vi "GenericPowerSupply.vi"() -> ()   [LabVIEW 2012]
uses:
  <userlib>/libdriver_powersupply/libdriver_powersupply.lvlib
panel:
  in  "SetCurrent":dbl step=0.2
  in  "ON/OFF":bool
  out "Current":dbl(graph)=10.19439697265625
  out "OPEN":bool
  out "NEG":bool
  out "POS":bool
  out "Alarm":bool
  out "Error":bool
  out "Standby":bool
  out "Operational":bool
  in  "stop":bool
  out "current out":dbl
  in  "Name":string="QUATTEST\u0000"
  in  "MDS":string="mdsserver:5000\u0000"
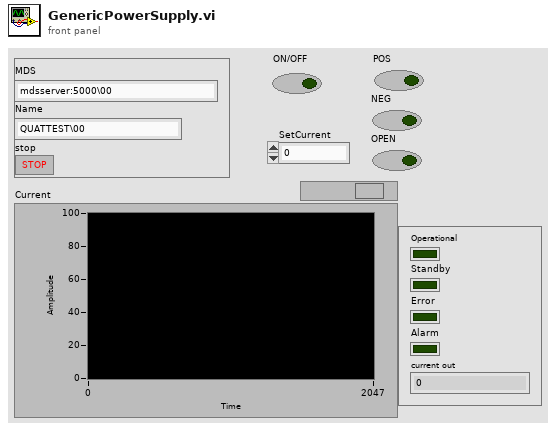
[diagram p1: front panel]
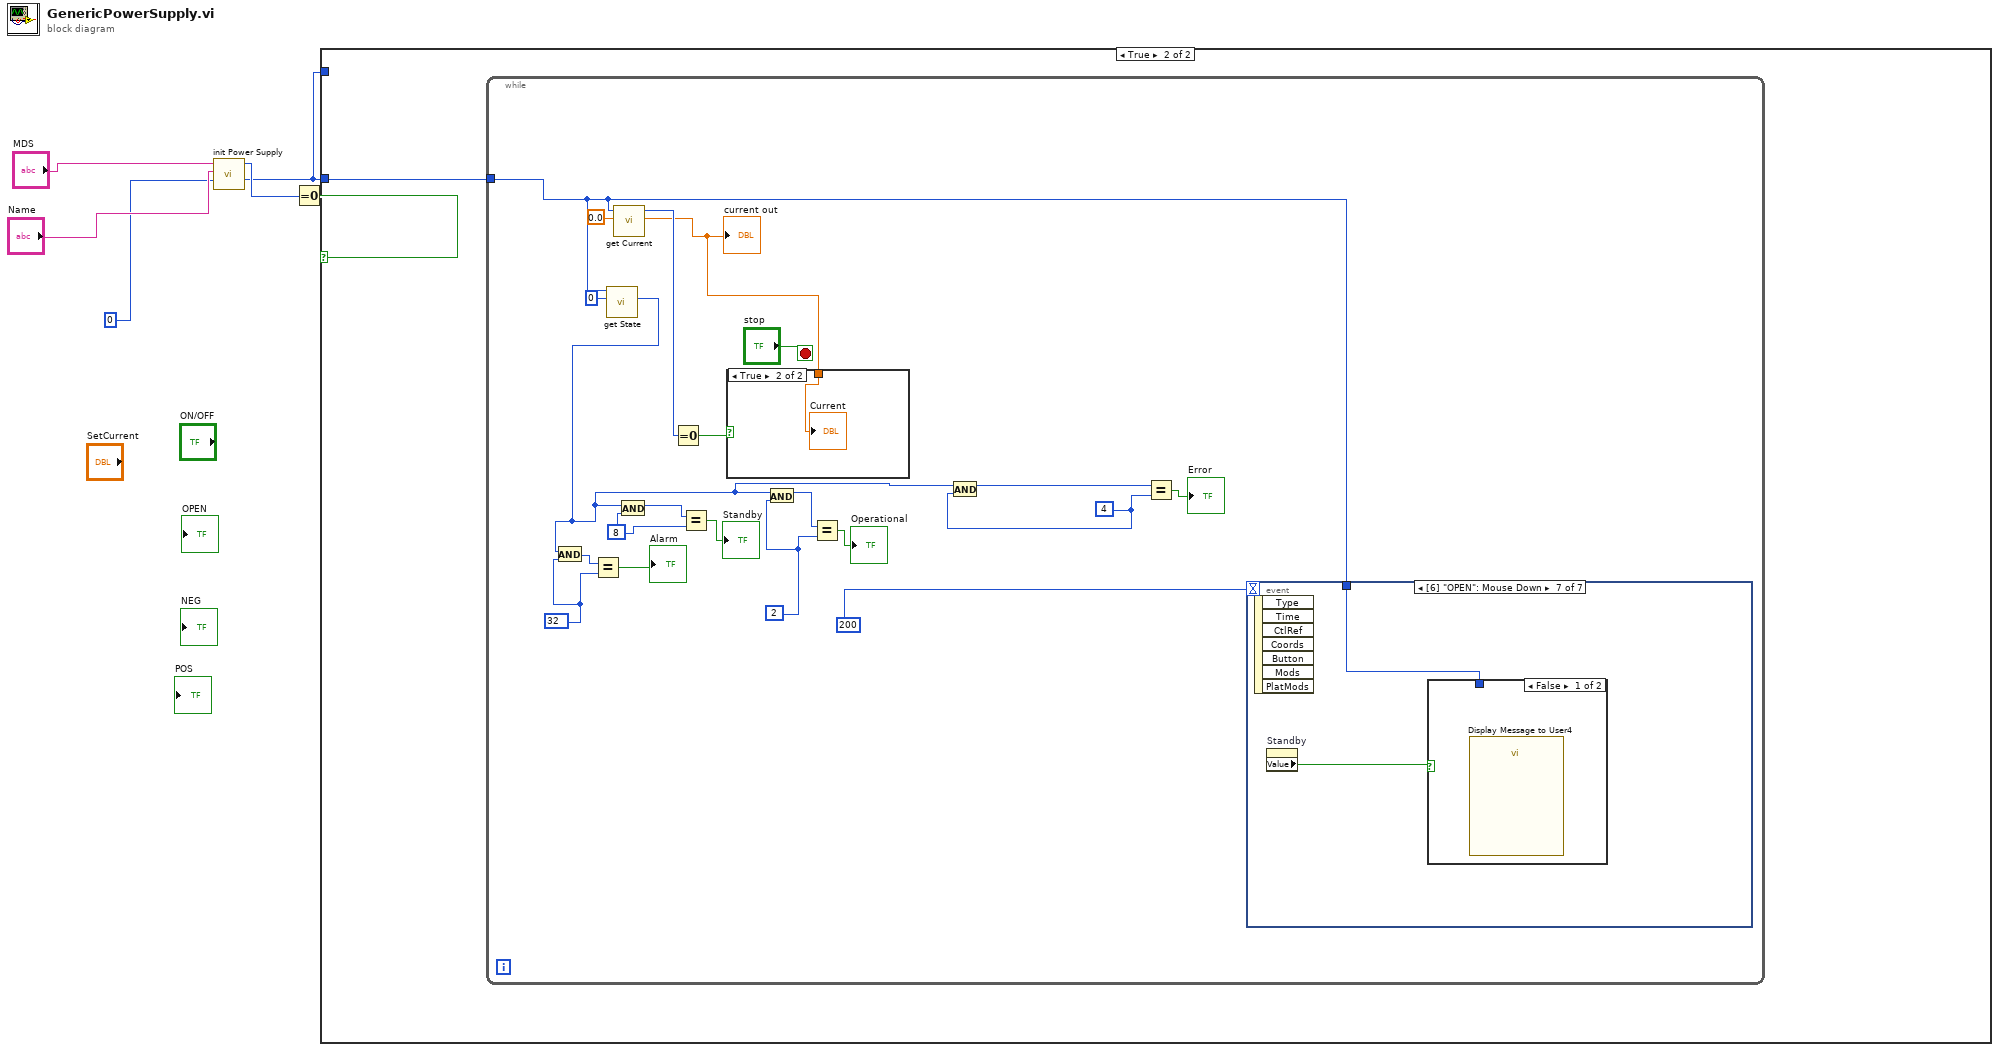
[diagram p0: block diagram]
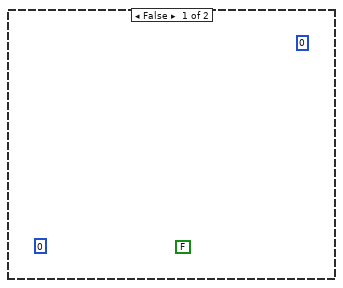
[diagram p2: hidden frame]
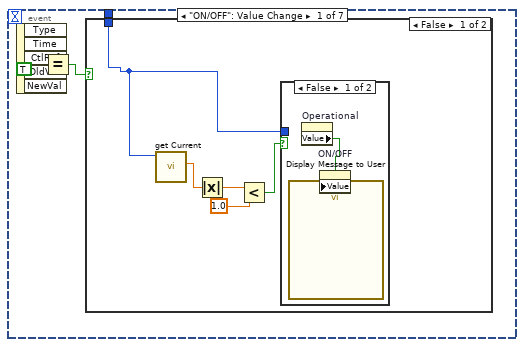
[diagram p3: hidden frame]
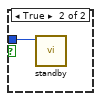
[diagram p4: hidden frame]
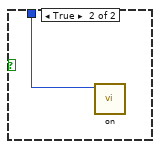
[diagram p5: hidden frame]
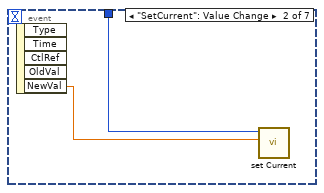
[diagram p6: hidden frame]
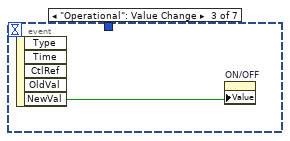
[diagram p7: hidden frame]
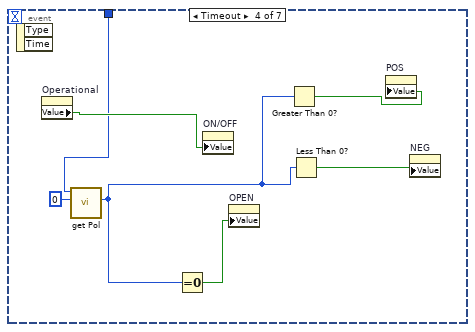
[diagram p8: hidden frame]
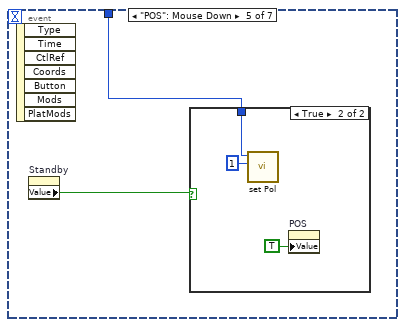
[diagram p9: hidden frame]
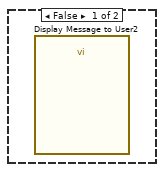
[diagram p10: hidden frame]
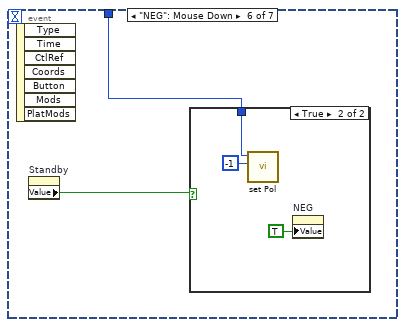
[diagram p11: hidden frame]
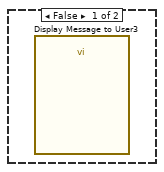
[diagram p12: hidden frame]
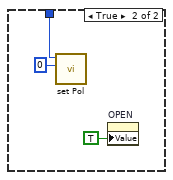
[diagram p13: hidden frame]
diagram:
  n1 = call <userlib>:"init Power Supply.vi"("devID"=u32 0 ("Numeric"), "name"="Name", "mds"="MDS") -> ("devID out"=w1:u32, "function return"=w3:i32)  [unwired: 7 in]
  n2 = Equal To 0?(x=w3) -> (x = 0?=w2:bool)
  n3 = case shown="True" w2 {
    tunnel: w1 -> [_ w7]
    tunnel: w1 -> [_ _]
    frame False {
      (unwired) 0 ("pol out")
      (unwired) 0 ("state out")
      (unwired) FALSE
    }
    frame True {
      n4 = while {
        tunnel: w7 -> [w17]
        stop <- "stop" stop-if-true
        w8 = u32 4 ("y")
        w11 = u32 2 ("y")
        w15 = u32 8 ("y")
        w13 = u32 32 ("y")
        n5 = call <userlib>:"get State.vi"("state"=0, "devID"=w17) -> ("state out"=w10:i32)  [unwired: 8 in, 1 out]
        n6 = And(x=w10, y=w13) -> (x .and. y?=w14:u32)
        n7 = Equal?(x=w14, y=w13) -> (x = y?=→"Alarm":bool)
        n8 = call <userlib>:"get Current.vi"("current"=0.0, "devID"=w17) -> ("current out"=w19:dbl, "function return"=w20:i32)  [unwired: 8 in]
        "current out" <- w19
        n9 = And(x=w10, y=w15) -> (x .and. y?=w16:u32)
        n10 = Equal To 0?(x=w20) -> (x = 0?=w21:bool)
        n11 = Equal?(x=w16, y=w15) -> (x = y?=→"Standby":bool)
        n12 = case shown="True" w21 {
          tunnel: w19 -> [_ w66]
          frame False {
          }
          frame True {
            "Current" <- w66
          }
        }
        n13 = And(x=w10, y=w11) -> (x .and. y?=w12:u32)
        n14 = Equal?(x=w12, y=w11) -> (x = y?=→"Operational":bool)
        n15 = And(x=w10, y=w8) -> (x .and. y?=w9:u32)
        n16 = Equal?(x=w9, y=w8) -> (x = y?=→"Error":bool)
        n17 = event shown="[6] \"OPEN\": Mouse Down" {
          selector: _ -> [_ _ _ _ _ _ _]
          dyn-events: _ -> [_ _ _ _ _ _ _]
          timeout: 200 -> [_ _ _ _ _ _ _]
          tunnel: w17 -> [w29 w42 _ w48 w52 w57 w62]
          event "ON/OFF": Value Change {
            n18 = event-data() -> ("NewVal"=w32:bool)  [unwired: 1 in, 4 out]
            n19 = Equal?(x=w32, y=TRUE) -> (x = y?=w30:bool)
            n20 = case shown="False" w30 {
              tunnel: w29 -> [w37 w40]
              frame False {
                n21 = call <userlib>:"get Current.vi"("devID"=w37) -> ("current out"=w36:dbl)  [unwired: 9 in, 1 out]
                n22 = Absolute Value(x=w36) -> (abs(x)=w35:dbl)
                n23 = Less?(x=w35, y=1.0) -> (x < y?=w33:bool)
                n24 = case shown="False" w33 {
                  tunnel: w37 -> [_ w39]
                  frame False {
                    n25 = call "Display Message to User"() -> ()  [unwired: 10 in, 2 out]
                    n26 = property on="Operational" class="Bool (strict)"() -> ("Value"=w38:bool)  [unwired: 2 in, 2 out]
                    n27 = property on="ON/OFF" class="Bool (strict)"("Value"=w38) -> ()  [unwired: 2 in, 2 out]
                  }
                  frame True {
                    n28 = call <userlib>:"standby.vi"("devID"=w39) -> ()  [unwired: 10 in, 1 out]
                  }
                }
              }
              frame True {
                n29 = call <userlib>:"on.vi"("devID"=w40) -> ()  [unwired: 10 in, 1 out]
              }
            }
          }
          event "SetCurrent": Value Change {
            n30 = event-data() -> ("NewVal"=w41:dbl)  [unwired: 1 in, 4 out]
            n31 = call <userlib>:"set Current.vi"("curr"=w41, "devID"=w42) -> ()  [unwired: 9 in, 1 out]
          }
          event "Operational": Value Change {
            n32 = event-data() -> ("NewVal"=w43:bool)  [unwired: 1 in, 4 out]
            n33 = property on="ON/OFF" class="Bool (strict)"("Value"=w43) -> ()  [unwired: 2 in, 2 out]
          }
          event Timeout {
            n34 = event-data() -> ()  [unwired: 1 in, 2 out]
            n35 = property on="Operational" class="Bool (strict)"() -> ("Value"=w50:bool)  [unwired: 2 in, 2 out]
            n36 = call <userlib>:"get Pol.vi"("pol"=0, "devID"=w48) -> ("pol out"=w45:i32)  [unwired: 8 in, 1 out]
            n37 = Equal To 0?(x=w45) -> (x = 0?=w47:bool)
            n38 = property on="ON/OFF" class="Bool (strict)"("Value"=w50) -> ()  [unwired: 2 in, 2 out]
            n39 = property on="OPEN" class="Bool (strict)"("Value"=w47) -> ()  [unwired: 2 in, 2 out]
            n40 = Greater Than 0?(x=w45) -> (x > 0?=w44:bool)
            n41 = Less Than 0?(x=w45) -> (x < 0?=w46:bool)
            n42 = property on="POS" class="Bool (strict)"("Value"=w44) -> ()  [unwired: 2 in, 2 out]
            n43 = property on="NEG" class="Bool (strict)"("Value"=w46) -> ()  [unwired: 2 in, 2 out]
          }
          event "POS": Mouse Down {
            n44 = event-data() -> ()  [unwired: 1 in, 7 out]
            n45 = property on="Standby" class="Bool (strict)"() -> ("Value"=w51:bool)  [unwired: 2 in, 2 out]
            n46 = case shown="True" w51 {
              tunnel: w52 -> [_ w54]
              frame False {
                n47 = call "Display Message to User2"() -> ()  [unwired: 10 in, 2 out]
              }
              frame True {
                n48 = call <userlib>:"set Pol.vi"("pol"=1, "devID"=w54) -> ()  [unwired: 9 in, 1 out]
                n49 = property on="POS" class="Bool (strict)"("Value"=TRUE ("POS")) -> ()  [unwired: 2 in, 2 out]
              }
            }
          }
          event "NEG": Mouse Down {
            n50 = event-data() -> ()  [unwired: 1 in, 7 out]
            n51 = property on="Standby" class="Bool (strict)"() -> ("Value"=w56:bool)  [unwired: 2 in, 2 out]
            n52 = case shown="True" w56 {
              tunnel: w57 -> [_ w59]
              frame False {
                n53 = call "Display Message to User3"() -> ()  [unwired: 10 in, 2 out]
              }
              frame True {
                n54 = call <userlib>:"set Pol.vi"("pol"=-1, "devID"=w59) -> ()  [unwired: 9 in, 1 out]
                n55 = property on="NEG" class="Bool (strict)"("Value"=TRUE ("NEG")) -> ()  [unwired: 2 in, 2 out]
              }
            }
          }
          event "OPEN": Mouse Down {
            n56 = event-data() -> ()  [unwired: 1 in, 7 out]
            n57 = property on="Standby" class="Bool (strict)"() -> ("Value"=w61:bool)  [unwired: 2 in, 2 out]
            n58 = case shown="False" w61 {
              tunnel: w62 -> [_ w64]
              frame False {
                n59 = call "Display Message to User4"() -> ()  [unwired: 10 in, 2 out]
              }
              frame True {
                n60 = call <userlib>:"set Pol.vi"("pol"=0, "devID"=w64) -> ()  [unwired: 9 in, 1 out]
                n61 = property on="OPEN" class="Bool (strict)"("Value"=TRUE ("OPEN")) -> ()  [unwired: 2 in, 2 out]
              }
            }
          }
        }
      }
    }
  }
